vi "UHR-Fleezers Control (host) - 12.0.vi"() -> ()   [LabVIEW 2012] (continued)
            n2040 = Unbundle By Name(w3404) -> ("Set 1"=w3403:dbl, "Set 2"=w3402:dbl)
            n2041 = Unbundle By Name(w3401) -> ("Set 1"=w3400:bool, "Set 2"=w3399:bool)
            n2042 = Select(t=w3397, s=w3400, f=w3403) -> (s? t:f=w3395:dbl)
            n2043 = Select(t=w3396, s=w3399, f=w3402) -> (s? t:f=w3394:dbl)
            n2044 = Bundle By Name(cluster=w3404, "Set 1"=w3395, "Set 2"=w3394) -> (w3392:cluster{"Set 1":dbl, "Set 2":dbl})
            n2045 = local write "Setpoints (V)"(w3392) -> ()
            n2046 = Multiply(x=3276.7, y=w3392) -> (x*y=w3393:cluster{"Set 1":dbl, "Set 2":dbl})
            n2047 = To Word Integer(number=w3393) -> (16bit integer=w3405:cluster{"Set 1":i16, "Set 2":i16})
          }
        }
        n2048 = Unbundle By Name(w3377) -> ("Set 1"=w3376:i16, "Set 2"=w3375:i16)
        n2049 = xnode "Read/Write Control"("FPGA VI Reference In"=w3373, "error in"=w3372, "FB Setpoint Set 1"=w3376, "FB Setpoint Set 2"=w3375) -> ("error out"=w3371:errorcluster)  [unwired: 1 out]
      }
      event "Invert GI": Value Change {
        n2050 = event-data() -> ()  [unwired: 7 out]
        n2051 = xnode "Read/Write Control"("FPGA VI Reference In"=w3410, "error in"=w3408, "Invert GI"="Invert GI", "Invert GI 2"="Invert GI") -> ("error out"=w3409:errorcluster)  [unwired: 1 out]
      }
      event "Green FB Setpoint (mV)", "Green FB Gains", "Green FB On/Off", "Current When FB OFF (%)", "Green int current ON count adj": Value Change {
        n2052 = event-data() -> ()  [unwired: 7 out]
        n2053 = local read "Green FB Setpoint (mV)"() -> (w3417:dbl)
        n2054 = local read "Current When FB OFF (%)"() -> (w3420:dbl)
        n2055 = Multiply(x=w3417, y=3.2767) -> (x*y=w3416:dbl)
        n2056 = Multiply(x=w3420, y=655.35) -> (x*y=w3421:dbl)
        n2057 = To Unsigned Word Integer(number=w3421) -> (unsigned 16bit integer=w3419:u16)
        n2058 = local read "Green int current ON count adj"() -> (w3424:u32)
        n2059 = local read "Green FB Gains"() -> (w3423:T14)
        n2060 = local read "Green Laser ON/Interlacing"() -> (w3414:bool)
        n2061 = local read "Green laser mode"() -> (w3413:enum32{"Laser ON", "Laser OFF", "Interlace"})
        n2062 = local read "Green FB On/Off"() -> (w3425:bool)
        n2063 = Equal?(x=w3413, y=enum32{"Laser ON", "Laser OFF", "Interlace"}."Interlace") -> (x = y?=w3411:bool)
        n2064 = Compound Arithmetic op=AND(w3411, w3425, w3414) -> (w3415:bool)
        n2065 = xnode "Read/Write Control"("FPGA VI Reference In"=w3428, "error in"=w3427, "Green FB Setpoint"=w3416, "Green FB On/Off"=w3415, "Current Out"=w3419, "Green int current ON count adj"=w3424, "Green FB Gains"=w3423) -> ("error out"=w3426:errorcluster)  [unwired: 1 out]
      }
      event "Green laser mode", "Green Laser ON/Interlacing": Value Change {
        n2066 = event-data() -> ()  [unwired: 7 out]
        n2067 = local write "Green Laser ON/OFF"("Green Laser ON/Interlacing") -> ()
        n2068 = case shown="True" "Green Laser ON/Interlacing" {
          tunnel: "Green laser mode" -> [_ w3442]
          tunnel: [enum32{"Laser ON", "Laser OFF", "Interlace"}."Laser OFF" ("Green laser mode") w3442] -> w3431
          tunnel: [FALSE w3438] -> w3430
          frame False {
          }
          frame True {
            n2069 = local read "Green FB On/Off"() -> (w3439:bool)
            n2070 = Equal?(x=w3442, y=enum32{"Laser ON", "Laser OFF", "Interlace"}."Interlace") -> (x = y?=w3440:bool)
            n2071 = And(x=w3440, y=w3439) -> (x .and. y?=w3438:bool)
          }
        }
        n2072 = xnode "Read/Write Control"("FPGA VI Reference In"=w3435, "error in"=w3433, "Operating Mode"=w3431, "Operating Mode 2"=w3431, "Green FB On/Off"=w3430) -> ("error out"=w3434:errorcluster)  [unwired: 1 out]
      }
      event "Green Laser ON/OFF": Value Change {
        n2073 = event-data() -> ()  [unwired: 7 out]
        n2074 = property on="Green Laser ON/Interlacing" class="Bool (strict)"("Val(Sgnl)"="Green Laser ON/OFF") -> ()  [unwired: 2 in, 2 out]
      }
      event "Test ttrig": Value Change {
        n2075 = event-data() -> ()  [unwired: 7 out]
        n2076 = xnode "Read/Write Control"("FPGA VI Reference In"=w3447, "error in"=w3446, "TTrig?"=TRUE) -> ("error out"=w3445:errorcluster)  [unwired: 1 out]
      }
      event "Neg. TTrig FPGA": Value Change {
        n2077 = event-data() -> ()  [unwired: 7 out]
        n2078 = xnode "Read/Write Control"("FPGA VI Reference In"=w3451, "error in"=w3450, "TTrig Negate Pos"="Neg. TTrig FPGA") -> ()  [unwired: 2 out]
      }
      event "- phase (APD 1 Gate)", "+ phase (APD 1 Gate)": Value Change {
        n2079 = event-data() -> ()  [unwired: 7 out]
        n2080 = local read "Phase Adj. (APD 1 Gate)"() -> (w3452:i16)
        n2081 = Negate(x=w3452) -> (-x=w3460:i16)
        n2082 = Select(t=w3460, s="- phase (APD 1 Gate)", f=w3452) -> (s? t:f=w3459:i16)
        n2083 = Or(x="- phase (APD 1 Gate)", y="+ phase (APD 1 Gate)") -> (x .or. y?=w3455:bool)
        n2084 = xnode "Read/Write Control"("FPGA VI Reference In"=w3462, "error in"=w3461, "Phase count adjustment (APD 1 Gate)"=w3459) -> ("FPGA VI Reference Out"=w3457:T19, "error out"=w3458:errorcluster)
        n2085 = xnode "Read/Write Control"("FPGA VI Reference In"=w3457, "error in"=w3458, "+ phase (APD 1 Gate)"=w3455) -> ("error out"=w3456:errorcluster)  [unwired: 1 out]
      }
      event "+ phase (APD 2 Gate)", "- phase (APD 2 Gate)": Value Change {
        n2086 = event-data() -> ()  [unwired: 7 out]
        n2087 = local read "Phase Adj. (APD 2 Gate)"() -> (w3463:i16)
        n2088 = Negate(x=w3463) -> (-x=w3471:i16)
        n2089 = Select(t=w3471, s="- phase (APD 2 Gate)", f=w3463) -> (s? t:f=w3470:i16)
        n2090 = Or(x="- phase (APD 2 Gate)", y="+ phase (APD 2 Gate)") -> (x .or. y?=w3466:bool)
        n2091 = xnode "Read/Write Control"("FPGA VI Reference In"=w3473, "error in"=w3472, "Phase count adjustment (APD 2 Gate)"=w3470) -> ("FPGA VI Reference Out"=w3468:T19, "error out"=w3469:errorcluster)
        n2092 = xnode "Read/Write Control"("FPGA VI Reference In"=w3468, "error in"=w3469, "+ phase (APD 2 Gate)"=w3466) -> ("error out"=w3467:errorcluster)  [unwired: 1 out]
      }
      event "Phase Adj. (APD Acq)", "+ phase (APD Acq)", "- phase (APD Acq)": Value Change {
        n2093 = event-data() -> ()  [unwired: 7 out]
        n2094 = local read "Phase Adj. (APD Acq)"() -> (w3476:i16)
        n2095 = Negate(x=w3476) -> (-x=w3482:i16)
        n2096 = Select(t=w3482, s="+ phase (APD Acq)", f=w3476) -> (s? t:f=w3481:i16)
        n2097 = Or(x="+ phase (APD Acq)", y="- phase (APD Acq)") -> (x .or. y?=w3477:bool)
        n2098 = xnode "Read/Write Control"("FPGA VI Reference In"=w3484, "error in"=w3483, "Phase Count Adjustment (APD Acq)"=w3481) -> ("FPGA VI Reference Out"=w3479:T19, "error out"=w3480:errorcluster)
        n2099 = xnode "Read/Write Control"("FPGA VI Reference In"=w3479, "error in"=w3480, "+ phase (APD Acq)"=w3477) -> ("error out"=w3478:errorcluster)  [unwired: 1 out]
      }
      event "Phase adj. (GI)", "+ phase (GI)", "- phase (GI)": Value Change {
        n2100 = event-data() -> ()  [unwired: 7 out]
        n2101 = Negate(x="Phase adj. (GI)") -> (-x=w3493:i16)
        n2102 = Select(t=w3493, s="+ phase (GI)", f="Phase adj. (GI)") -> (s? t:f=w3492:i16)
        n2103 = Or(x="+ phase (GI)", y="- phase (GI)") -> (x .or. y?=w3488:bool)
        n2104 = xnode "Read/Write Control"("FPGA VI Reference In"=w3495, "error in"=w3494, "Phase count adjustment (GI)"=w3492) -> ("FPGA VI Reference Out"=w3490:T19, "error out"=w3491:errorcluster)
        n2105 = xnode "Read/Write Control"("FPGA VI Reference In"=w3490, "error in"=w3491, "+ phase (GI)"=w3488) -> ("error out"=w3489:errorcluster)  [unwired: 1 out]
      }
      event "Phase adj. (GI) 2", "+ phase (GI) 2", "- phase (GI) 2": Value Change {
        n2106 = event-data() -> ()  [unwired: 7 out]
        n2107 = Negate(x="Phase adj. (GI) 2") -> (-x=w3504:i16)
        n2108 = Select(t=w3504, s="+ phase (GI) 2", f="Phase adj. (GI) 2") -> (s? t:f=w3503:i16)
        n2109 = Or(x="+ phase (GI) 2", y="- phase (GI) 2") -> (x .or. y?=w3499:bool)
        n2110 = xnode "Read/Write Control"("FPGA VI Reference In"=w3506, "error in"=w3505, "Phase count adjustment (GI) 2"=w3503) -> ("FPGA VI Reference Out"=w3501:T19, "error out"=w3502:errorcluster)
        n2111 = xnode "Read/Write Control"("FPGA VI Reference In"=w3501, "error in"=w3502, "+ phase (GI) 2"=w3499) -> ("error out"=w3500:errorcluster)  [unwired: 1 out]
      }
      event "Phase adj. (Green FB)", "- phase (Green FB)", "+ phase (Green FB)": Value Change {
        n2112 = event-data() -> ()  [unwired: 7 out]
        n2113 = Negate(x="Phase adj. (Green FB)") -> (-x=w3515:i16)
        n2114 = Select(t=w3515, s="+ phase (Green FB)", f="Phase adj. (Green FB)") -> (s? t:f=w3514:i16)
        n2115 = Or(x="+ phase (Green FB)", y="- phase (Green FB)") -> (x .or. y?=w3510:bool)
        n2116 = xnode "Read/Write Control"("FPGA VI Reference In"=w3517, "error in"=w3516, "Phase count adjustment (Green FB)"=w3514) -> ("FPGA VI Reference Out"=w3512:T19, "error out"=w3513:errorcluster)
        n2117 = xnode "Read/Write Control"("FPGA VI Reference In"=w3512, "error in"=w3513, "+ phase (Green FB)"=w3510) -> ("error out"=w3511:errorcluster)  [unwired: 1 out]
      }
      event "Invert APD Gate", "APD Gate ON Count", "APD Gate OFF Count", "APD Gate", "APD Integration Time (s)", "APD 1 AO Mult.", "APD 2 AO Mult.", "On one out of X cycles": Value Change {
        n2118 = event-data() -> ()  [unwired: 7 out]
        n2119 = Add(x="GI Frequency, ON count", y="GI Frequency, OFF count") -> (x+y=w3521:u32)
        n2120 = Add(x="APD Gate ON Count", y="APD Gate OFF Count") -> (x+y=w3534:u32)
        n2121 = Multiply(x="On one out of X cycles", y=w3521) -> (x*y=w3518:u32)
        "Green FB Count" <- w3518
        n2122 = Subtract(x=w3518, y="GI Frequency, ON count") -> (x-y=w3519:u32)
        n2123 = Multiply(x=w3534, y="On one out of X cycles") -> (x*y=w3533:u32)
        n2124 = Subtract(x=w3533, y="APD Gate ON Count") -> (x-y=w3532:u32)
        n2125 = local read "DMA Update Period (s)"() -> (w3535:dbl)
        n2126 = Multiply(x="APD Integration Time (s)", y=40000000.0) -> (x*y=w3540:dbl)
        n2127 = Reciprocal(x="APD Integration Time (s)") -> (1/x=→"APD Acq Rate (Hz)":dbl)
        n2128 = To Unsigned Long Integer(number=w3540) -> (unsigned 32bit integer=w3524:u32)
        "APD Int. Count" <- w3524
        n2129 = xnode "Read/Write Control"("FPGA VI Reference In"=w3544, "error in"=w3543, "Invert APD Gate"="Invert APD Gate", "APD Gate ON Count"="APD Gate ON Count", "APD Gate OFF Count"=w3532, "APD Acq Rate Count"=w3524, "APD Gate Operating Mode"="APD Gate", "APD 1 AO scale factor"="APD 1 AO Mult.", "APD 2 AO scale factor"="APD 2 AO Mult.", "Green interlace ON count"="GI Frequency, ON count", "Green interlace OFF count"=w3519, "Green interlace ON count 2"="GI Frequency, ON count", "Green interlace OFF count 2"=w3519, "Green FB Count"=w3518) -> ("error out"=w3542:errorcluster)  [unwired: 1 out]
        n2130 = Divide(x=w3535, y="APD Integration Time (s)") -> (x/y=w3538:dbl)
        n2131 = Multiply(x=2.0, y=w3538) -> (x*y=w3537:dbl)
        n2132 = local write "APD Samples/FIFO Acq."(w3538) -> ()
        n2133 = local write "APD Elements/DMA read"(w3537) -> ()
      }
      event "Number of F/B Scans (AOD)", "Scan Speed (nm/s)", "Scan BD", "Initial delta (MHz)", "Step Size (nm)", "Scan Range (nm)": Value Change {
        w3606 = 123.0  # AOM cal (nm/MHz)
        n2134 = event-data() -> ()  [unwired: 7 out]
        n2135 = local read "BD 1 Frequency 1 (MHz)"() -> (w3589:dbl)
        n2136 = local read "AOM X Cal (nm/MHz)"() -> (w3581:dbl)
        n2137 = local read "X RF Frequency Limits (MHz)"() -> (w3593:T16)
        n2138 = local read "Y RF Frequency Limits (MHz)"() -> (w3590:T16)
        n2139 = local read "BD 2 Frequency 1 (MHz)"() -> (w3595:dbl)
        n2140 = Negate(x="Scan Range (nm)") -> (-x=w3559:dbl)
        n2141 = Divide(x=w3559, y=w3581) -> (x/y=w3563:dbl)
        n2142 = Select(t=w3593, s="Scan BD", f=w3590) -> (s? t:f=w3592:T16)
        n2143 = Select(t=w3589, s="Scan BD", f=w3595) -> (s? t:f=w3594:dbl)
        n2144 = Unbundle By Name(w3592) -> ("Maximum"=w3601:dbl, "Minimum"=w3600:dbl)
        n2145 = Add(x=w3563, y=w3594) -> (x+y=w3598:dbl)
        n2146 = Divide(x=w3559, y="Step Size (nm)") -> (x/y=w3578:dbl)
        n2147 = Divide(x="Step Size (nm)", y=w3581) -> (x/y=w3587:dbl)
        n2148 = Absolute Value(x=w3578) -> (abs(x)=w3562:dbl)
        n2149 = Sign(1:w3559) -> (0:w3560:dbl)
        n2150 = In Range and Coerce(upper limit=w3601, x=w3598, lower limit=w3600) -> (coerced(x)=w3597:dbl, In Range?=w3599:bool)
        n2151 = To Unsigned Quad Integer(1:w3562) -> (0:w3577:u64)
        "Scan steps (AOD)" <- w3577
        n2152 = call "IR AOM freq to word.vi"("Frequency In (MHz)"=w3587) -> ("Frequency Word Out (double)"=w3584:dbl)
        n2153 = Multiply(x=w3560, y=w3584) -> (x*y=w3561:dbl)
        n2154 = Subtract(x=w3598, y=w3597) -> (x-y=w3596:dbl)
        n2155 = To Quad Integer(1:w3561) -> (0:w3583:i64)
        "Incr. int (AOD)" <- w3583
        n2156 = Subtract(x=w3563, y=w3596) -> (x-y=w3582:dbl)
        "Scan Range (MHz)" <- w3582
        n2157 = Select(t=w3563, s=w3599, f=w3582) -> (s? t:f=w3602:dbl)
        n2158 = Multiply(x=w3582, y=w3581) -> (x*y=w3580:dbl)
        n2159 = Decrement(x=w3577) -> (x-1=w3630:u64)
        n2160 = Negate(x=w3580) -> (-x=w3576:dbl)
        n2161 = local write "Scan Range (nm)"(w3576) -> ()
        n2162 = Divide(x=w3602, y=w3630) -> (x/y=w3586:dbl)
        "Scan Increment (MHz)" <- w3586
        n2163 = call "IR AOM freq to word.vi"("Frequency In (MHz)"=w3586) -> ("Frequency Word Out (double)"=w3585:dbl)
        n2164 = Divide(x="Step Size (nm)", y="Scan Speed (nm/s)") -> (x/y=w3573:dbl)
        n2165 = To Quad Integer(1:w3585) -> ()  [unwired: 1 out]
        n2166 = local read "Number Interlace Sets"() -> (w3557:u8)
        n2167 = local read "AI Count (ticks)"() -> (w3558:u32)
        n2168 = local read "Total Counts (ticks)"() -> (w3556:u32)
        n2169 = local read "# Samples/trap"() -> (w3588:u32)
        n2170 = Multiply(x=w3558, y=w3557) -> (x*y=w3555:u32)
        n2171 = Divide(x=w3556, y=w3555) -> (x/y=w3554:dbl)
        n2172 = Select(t=w3589, s="Scan BD", f=w3595) -> (s? t:f=w3627:dbl)
        "Initial freq. (MHz)" <- w3627
        n2173 = Add(x=w3602, y=w3627) -> (x+y=→"Final freq. (MHz)":dbl)
        n2174 = Divide(x=w3556, y=40000000.0) -> (x/y=w3572:dbl)
        n2175 = Divide(x=w3573, y=w3572) -> (x/y=w3571:dbl)
        n2176 = To Unsigned Quad Integer(1:w3571) -> (0:w3546:u64)
        n2177 = Quotient & Remainder(x=w3546, y=u64 2) -> (x-y*floor(x/y)=w3550:u64)  [unwired: 1 out]
        n2178 = Equal?(x=w3550, y=u64 0) -> (x = y?=w3548:bool)
        n2179 = Decrement(x=w3546) -> (x-1=w3547:u64)
        n2180 = Select(t=w3546, s=w3548, f=w3547) -> (s? t:f=w3545:u64)
        "Cycles/step (AOD)" <- w3545
        n2181 = xnode "Read/Write Control"("FPGA VI Reference In"=w3638, "error in"=w3637, "Scan steps"=w3577, "Number of scans"="Number of F/B Scans (AOD)", "Cycles per step"=w3545, "Scan freq.  increment"=w3583, "Scan BD"="Scan BD") -> ("error out"=w3636:errorcluster)  [unwired: 1 out]
        n2182 = Multiply(x=w3577, y=w3545) -> (x*y=w3631:u64)
        n2183 = Multiply(x=w3631, y=u64 2) -> (x*y=w3553:u64)
        n2184 = Multiply(x=w3554, y=w3553) -> (x*y=w3552:dbl)
        "Data points/scan (f/b)" <- w3552
        n2185 = Multiply(x=w3552, y="Number of F/B Scans (AOD)") -> (x*y=w3634:dbl)
        "Data points/scans" <- w3634
        n2186 = Divide(x=w3634, y=w3588) -> (x/y=→"N sets should be saved":dbl)
        n2187 = Multiply(x=w3631, y=w3572) -> (x*y=w3570:dbl)
        "Time/Scan (s) (AOD)" <- w3570
        n2188 = Select(t=w3602, s="Scan BD", f=0.0) -> (s? t:f=w3628:dbl)
        n2189 = Select(t=0.0, s="Scan BD", f=w3602) -> (s? t:f=w3624:dbl)
        n2190 = local read "BD 2 Frequency 2 (MHz)"() -> (w3620:dbl)
        n2191 = local read "BD 1 Frequency 2 (MHz)"() -> (w3623:dbl)
        n2192 = Add(x=w3624, y=w3595) -> (x+y=w3621:dbl)
        n2193 = Add(x=w3589, y=w3628) -> (x+y=w3622:dbl)
        n2194 = Multiply(x=w3570, y=2.0) -> (x*y=w3569:dbl)
        n2195 = Multiply(x=w3569, y="Number of F/B Scans (AOD)") -> (x*y=w3566:dbl)
        n2196 = Divide(x=w3566, y=60.0) -> (x/y=→"Time to Finish All (min)":dbl)
        n2197 = Add(x="Trap 2 Bead Size (nm)", y="Trap 1 Bead Size (nm)") -> (x+y=w3610:dbl)
        n2198 = Divide(x=w3610, y=2.0) -> (x/y=w3604:dbl)
        n2199 = local read "Initial delta (MHz)"() -> (w3607:dbl)
        n2200 = Subtract(x=w3621, y=w3620) -> (x-y=w3618:dbl)
        n2201 = Subtract(x=w3622, y=w3623) -> (x-y=w3619:dbl)
        n2202 = Square(x=w3618) -> (x^2=w3617:dbl)
        n2203 = Square(x=w3619) -> (x^2=w3616:dbl)
        n2204 = Add(x=w3616, y=w3617) -> (x+y=w3615:dbl)
        n2205 = Square Root(x=w3615) -> (sqrt(x)=w3614:dbl)
        "Final delta (MHz)" <- w3614
        n2206 = Multiply(x=w3606, y=w3614) -> (x*y=w3613:dbl)
        n2207 = Multiply(x=w3607, y=w3606) -> (x*y=w3605:dbl)
        n2208 = Subtract(x=w3605, y=w3604) -> (x-y=→"Initial sep (nm)":dbl)
        n2209 = Subtract(x=w3613, y=w3604) -> (x-y=→"Final sep (nm)":dbl)
      }
      event "Freq or Amp switch first", "Swap F1 and F2", "Freq switch delay", "Amp switch delay": Value Change {
        n2210 = event-data() -> ()  [unwired: 7 out]
        n2211 = local read "Freq or Amp switch first"() -> (w3639:bool)
        n2212 = local read "Amp switch delay"() -> (w3640:u16)
        n2213 = local read "Freq switch delay"() -> (w3642:u16)
        n2214 = local read "Swap F1 and F2"() -> (w3641:bool)
        n2215 = xnode "Read/Write Control"("FPGA VI Reference In"=w3645, "error in"=w3644, "Freq switch delay"=w3642, "Swap F1 and F2"=w3641, "Amp switch delay"=w3640, "Freq or Amp switch first"=w3639) -> ("error out"=w3643:errorcluster)  [unwired: 1 out]
      }
      event "Scan steps (MCL)", "Number of scans (MCL)", "Scan Range (V)\n(of steps)", "2D or 1D Scan", "N APD Samp/step", "Fast Scan Dir", "Continuous MCL Scanning", "Scan lines (y)": Value Change {
        w3647 = 32767.0 ("y")
        n2216 = event-data() -> ()  [unwired: 7 out]
        n2217 = Select(t="Scan lines (y)", s="2D or 1D Scan", f="Number of scans (MCL)") -> (s? t:f=w3652:u64)
        n2218 = Decrement(x="Scan steps (MCL)") -> (x-1=w3668:u64)
        n2219 = Divide(x="Scan Range (V)\n(of steps)", y=w3668) -> (x/y=w3667:dbl)
        "Desired Scan Incr (V)" <- w3667
        n2220 = local read "APD Integration Time (s)"() -> (w3660:dbl)
        n2221 = Multiply(x=w3667, y=w3647) -> (x*y=w3676:dbl)
        n2222 = Divide(x=w3676, y=10.0) -> (x/y=w3666:dbl)
        "Desired incr (int)" <- w3666
        n2223 = local read "Update Count (MCL)"() -> (w3672:u32)
        n2224 = Round Toward -Infinity(1:w3666) -> (0:w3675:dbl)
        n2225 = To Word Integer(number=w3675) -> (16bit integer=w3650:i16)
        "Actual Incr. int (MCL)" <- w3650
        n2226 = Multiply(x=w3660, y=40000000.0) -> (x*y=w3673:dbl)
        n2227 = Divide(x=w3673, y=w3672) -> (x/y=w3671:dbl)
        n2228 = Multiply(x=i16 10, y=w3650) -> (x*y=w3648:i16)
        n2229 = Multiply(x="N APD Samp/step", y=w3671) -> (x*y=w3670:dbl)
        "Cycles/step (MCL)" <- w3670
        n2230 = Divide(x=w3648, y=w3647) -> (x/y=→"Actual MCL Inc (V)":dbl)
        n2231 = Multiply(x="N APD Samp/step", y="Scan steps (MCL)") -> (x*y=w3662:dbl)
        n2232 = local read "APD Samples/FIFO Acq."() -> (w3659:dbl)
        n2233 = Multiply(x=w3662, y=u64 2) -> (x*y=w3661:dbl)
        "Data points/scan (f+b)" <- w3661
        n2234 = Multiply(x=w3661, y=w3652) -> (x*y=w3679:dbl)
        "Data points/scans (MCL)" <- w3679
        n2235 = Multiply(x=w3660, y=w3661) -> (x*y=w3653:dbl)
        "Time/f+b scan (s) (MCL)" <- w3653
        n2236 = Divide(x=w3679, y=w3659) -> (x/y=→"N sets should be saved (MCL)":dbl)
        n2237 = Multiply(x=w3653, y=w3652) -> (x*y=→"Total Time (s)":dbl)
        n2238 = Not(x="Fast Scan Dir") -> (.not. x?=w3657:bool)
        n2239 = xnode "Read/Write Control"("FPGA VI Reference In"=w3683, "error in"=w3682, "Scan steps (MCL)"="Scan steps (MCL)", "Number of scans (MCL)"=w3652, "Cycles per step (MCL)"=w3670, "Scan freq.  increment (MCL)"=w3650, "1D or 2D Scan?"="2D or 1D Scan", "MCL Scan Axis"=w3657, "Cont. Scan (MCL)"="Continuous MCL Scanning") -> ("error out"=w3681:errorcluster)  [unwired: 1 out]
      }
      event "Read Cal": Value Change {
        w3685 = 1000.0 ("y")
        n2240 = event-data() -> ()  [unwired: 7 out]
        n2241 = local read "Save file name"() -> (w3710:path)
        n2242 = local write "Read Cal"(FALSE ("Read Cal")) -> ()
        n2243 = Strip Path(path=w3710) -> (stripped path=w3709:path)  [unwired: 1 out]
        n2244 = Path To String(path=w3709) -> (string=w3708:string)
        n2245 = Concatenate Strings(w3708, "\\current.cal" ("string")) -> (w3706:string)
        n2246 = String To Path(string=w3706) -> (path=w3705:path)
        n2247 = Open/Create/Replace File(file path (use dialog)=w3705, operation (0:open)=T35."open", access (0:read/write)=enum16{"read/write", "read-only", "write-only"}."read-only") -> (refnum out=w3713:refnum<file>, error out=w3699:errorcluster)  [unwired: 1 in, 3 out]
        n2248 = Deny Access(4:w3699, 7:w3713) -> (0:w3698:errorcluster, 3:w3704:refnum<file>)  [unwired: 1 out]
        n2249 = Read from Binary File(5:0.0, 8:w3698, 9:T36."big-endian, network order" ("byte order (0:big-endian, network order)"), 10:-1 ("count (1)"), 11:w3704) -> (0:w3697:errorcluster, 2:w3695:dbl[], 3:w3700:refnum<file>)  [unwired: 2 out]
        n2250 = Array To Cluster(array=w3695) -> (cluster=w3694:T44)
        n2251 = Unbundle(w3694) -> ("[0]"=w3693:dbl, "[1]"=w3692:dbl, "[2]"=w3691:dbl, "[3]"=w3690:dbl, "[4]"=w3689:dbl, "[5]"=w3688:dbl)
        n2252 = Close File(refnum=w3700, error in=w3697) -> (error out=→"Read cal error":errorcluster)  [unwired: 1 out]
        n2253 = Multiply(x=w3688, y=w3685) -> (x*y=w3686:dbl)
        n2254 = local write "T2 kappa_x (pN/nm)"(w3690) -> ()
        n2255 = local write "T1 kappa_x (pN/nm)"(w3691) -> ()
        n2256 = local write "T1 alpha_x (nm/V)"(w3693) -> ()
        n2257 = local write "T2 alpha_x (nm/V)"(w3692) -> ()
        n2258 = Multiply(x=w3689, y=w3685) -> (x*y=w3687:dbl)
        n2259 = local write "T1 offset_x (mV)"(w3687) -> ()
        n2260 = local write "T2 offset_x (mV)"(w3686) -> ()
      }
      event "Abort MCL Scan": Value Change {
        n2261 = event-data() -> ()  [unwired: 7 out]
        n2262 = local write "MCL Scanning"(FALSE ("MCL Scanning")) -> ()
        n2263 = xnode "Read/Write Control"("FPGA VI Reference In"=w3718, "error in"=w3717, "Abort scan (MCL)"="Abort MCL Scan") -> ("error out"=w3716:errorcluster)  [unwired: 1 out]
      }
      event "Update Count (MCL)": Value Change {
        n2264 = event-data() -> ()  [unwired: 7 out]
        n2265 = xnode "Read/Write Control"("FPGA VI Reference In"=w3722, "error in"=w3721, "MCL count"="Update Count (MCL)") -> ("error out"=w3720:errorcluster)  [unwired: 1 out]
      }
      event "Phase adjust (MCL)", "+ phase (MCL)", "- phase (MCL)": Value Change {
        n2266 = event-data() -> ()  [unwired: 7 out]
        n2267 = Negate(x="Phase adjust (MCL)") -> (-x=w3731:i16)
        n2268 = Select(t=w3731, s="- phase (MCL)", f="Phase adjust (MCL)") -> (s? t:f=w3729:i16)
        n2269 = Or(x="- phase (MCL)", y="+ phase (MCL)") -> (x .or. y?=w3724:bool)
        n2270 = xnode "Read/Write Control"("FPGA VI Reference In"=w3733, "error in"=w3732, "Phase count adjustment (MCL)"=w3729) -> ("FPGA VI Reference Out"=w3725:T19, "error out"=w3726:errorcluster)
        n2271 = xnode "Read/Write Control"("FPGA VI Reference In"=w3725, "error in"=w3726, "+ phase (MCL)"=w3724) -> ("error out"=w3723:errorcluster)  [unwired: 1 out]
      }
      event "Abort AOD Scan": Value Change {
        n2272 = event-data() -> ()  [unwired: 7 out]
        n2273 = xnode "Read/Write Control"("FPGA VI Reference In"=w3737, "error in"=w3736, "Abort scan"="Abort AOD Scan") -> ("error out"=w3735:errorcluster)  [unwired: 1 out]
      }
      event "Continuous AOD Scanning": Value Change {
        n2274 = event-data() -> ()  [unwired: 7 out]
        n2275 = xnode "Read/Write Control"("FPGA VI Reference In"=w3741, "error in"=w3740, "Cont. Scan"="Continuous AOD Scanning") -> ("error out"=w3739:errorcluster)  [unwired: 1 out]
      }
      event "Index": Value Change {
        n2276 = event-data() -> ()  [unwired: 7 out]
        n2277 = call "Create new save file.vi"("Insert"="", "Ext"=".dat" ("string"), "Index In"="Index") -> ("Path Out"=→"Save file name":path, "Index Out"=w3742:dbl)
        "Save index" <- w3742
        n2278 = local write "Index"(w3742) -> ()
      }
      event "AO1", "AO2": Value Change {
        w3757 = 10.0 ("y")
        w3756 = 32767.0 ("y")
        n2279 = event-data() -> ()  [unwired: 7 out]
        n2280 = local read "AO2"() -> (w3755:dbl)
        n2281 = local read "AO1"() -> (w3752:dbl)
        n2282 = Multiply(x=w3752, y=w3756) -> (x*y=w3751:dbl)
        n2283 = Multiply(x=w3755, y=w3756) -> (x*y=w3754:dbl)
        n2284 = Divide(x=w3751, y=w3757) -> (x/y=w3750:dbl)
        n2285 = Divide(x=w3754, y=w3757) -> (x/y=w3753:dbl)
        n2286 = To Word Integer(number=w3750) -> (16bit integer=w3758:i16)
        n2287 = To Word Integer(number=w3753) -> (16bit integer=w3759:i16)
        n2288 = xnode "Read/Write Control"("FPGA VI Reference In"=w3749, "error in"=w3748, "AO1"=w3758, "AO2"=w3759) -> ("error out"=w3747:errorcluster)  [unwired: 1 out]
      }
      event "Inject Pump 1": Value Change {
        n2289 = event-data() -> ()  [unwired: 7 out]
        n2290 = local read "Use Harvard pumps\nfor beads (else Chemyx)"() -> (w3761:bool)
        n2291 = case shown="True" w3761 {
          tunnel: "Inject Pump 1" -> [w3765 w3803]
          tunnel: w3760 -> [_ w3804]
          frame False {
            n2292 = local read "Pump write delay (ms)"() -> (w3764:dbl)
            n2293 = local read "Chemyx Syringe Pump Serial Port"() -> (w3763:refnum<visa-resource-name>)
            n2294 = case shown="True" w3765 {
              tunnel: w3764 -> [w3771 w3785]
              tunnel: w3763 -> [w3768 w3784]
              frame False {
                n2295 = flat-sequence {
                  tunnel: w3768 -> [w3772]
                  tunnel: [w3772] -> w3769
                  tunnel: w3771 -> [_]
                  tunnel: [w3775] -> w3770
                  tunnel: w3769 -> [w3775]
                  tunnel: w3770 -> [w3776]
                  tunnel: [w3776] -> w3766
                  tunnel: [w3778] -> w3767
                  tunnel: w3766 -> [w3778]
                  tunnel: w3767 -> [w3780]
                  frame #0 {
                    n2296 = call "Write to pump.vi"("string"="enter pump1", "VISA resource name"=w3772) -> ()  [unwired: 1 out]
                  }
                  frame #1 {
                    n2297 = Wait (ms)(milliseconds to wait="Pump pause delay (ms)") -> ()  [unwired: 1 out]
                  }
                  frame #2 {
                    n2298 = call "Write to pump.vi"("string"="stop", "VISA resource name"=w3776) -> ()  [unwired: 1 out]
                  }
                  frame #3 {
                    n2299 = Wait (ms)(milliseconds to wait=u32 500) -> ()  [unwired: 1 out]
                  }
                  frame #4 {
                    n2300 = call "Write to pump.vi"("string"="stop", "VISA resource name"=w3780) -> ()  [unwired: 1 out]
                  }
                }
              }
              frame True {
                n2301 = flat-sequence {
                  tunnel: w3784 -> [w3794]
                  tunnel: w3785 -> [w3789]
                  tunnel: w3785 -> [w3796]
                  tunnel: w3784 -> [w3797]
                  tunnel: [w3797] -> w3782
                  tunnel: [w3799] -> w3783
                  tunnel: w3782 -> [w3799]
                  tunnel: w3783 -> [w3801]
                  frame #0 {
                    n2302 = local read "All Pump Parameters"() -> (w3788:T5)
                    n2303 = Unbundle By Name(w3788) -> ("Pump 1"=w3795:T45)
                    n2304 = call "Set pump parameters.vi"("Pump write delay (ms)"=w3789, "Volume (uL)"="Ch 1 Inject Volume (uL)", "Rate (uL/h)"="Ch 1 Inject Rate (ul/h)", "Units"=4.0, "Pump #"=1.0, "Pump Parameters In"=w3795, "VISA resource name"=w3794) -> ("Pump Parameters Out"=w3787:T45)  [unwired: 3 in]
                    n2305 = Bundle By Name(cluster=w3788, "Pump 1"=w3787) -> (w3786:T5)
                    n2306 = local write "All Pump Parameters"(w3786) -> ()
                  }
                  frame #1 {
                    n2307 = Wait (ms)(milliseconds to wait=w3796) -> ()  [unwired: 1 out]
                  }
                  frame #2 {
                    n2308 = call "Write to pump.vi"("string"="start", "VISA resource name"=w3797) -> ()  [unwired: 1 out]
                  }
                  frame #3 {
                    n2309 = Wait (ms)(milliseconds to wait=u32 500) -> ()  [unwired: 1 out]
                  }
                  frame #4 {
                    n2310 = call "Write to pump.vi"("string"="start", "VISA resource name"=w3801) -> ()  [unwired: 1 out]
                  }
                }
              }
            }
          }
          frame True {
            n2311 = case shown="False" w3803 {
              tunnel: w3804 -> [w3805 w3815]
              frame False {
                n2312 = flat-sequence {
                  tunnel: w3805 -> [w3807]
                  frame #0 {
                    n2313 = local write "Flushing P1"(FALSE ("Flushing P1")) -> ()
                    n2314 = Concatenate Strings("stop" ("string"), "\r") -> (w3809:string)
                    n2315 = VISA Write(VISA resource name=w3807, write buffer=w3809) -> ()  [unwired: 1 in, 3 out]
                  }
                  frame #1 {
                    n2316 = property on="Clear Volume P1" class="Bool (strict)"("Val(Sgnl)"=TRUE ("Value (Signaling)")) -> ()  [unwired: 2 in, 2 out]
                  }
                }
              }
              frame True {
                n2317 = local read "Normal Flow Rate (ul/h) P1"() -> (w3813:dbl)
                n2318 = Number To Decimal String(number=w3813) -> (decimal integer string=w3819:string)  [unwired: 1 in]
                n2319 = Concatenate Strings("irate  " ("string"), w3819, " u/h" ("string"), "\r") -> (w3817:string)
                n2320 = VISA Write(VISA resource name=w3815, write buffer=w3817) -> (VISA resource name out=w3814:refnum<visa-resource-name>)  [unwired: 1 in, 2 out]
                n2321 = Concatenate Strings("irun" ("string"), "\r") -> (w3821:string)
                n2322 = VISA Write(VISA resource name=w3814, write buffer=w3821) -> ()  [unwired: 1 in, 3 out]
              }
            }
          }
        }
      }
      event "Inject Pump 3": Value Change {
        n2323 = event-data() -> ()  [unwired: 7 out]
        n2324 = local read "Use Harvard pumps\nfor beads (else Chemyx)"() -> (w3824:bool)
        n2325 = case shown="True" w3824 {
          tunnel: "Inject Pump 3" -> [w3828 w3867]
          tunnel: w3823 -> [_ w3866]
          frame False {
            n2326 = local read "Pump write delay (ms)"() -> (w3827:dbl)
            n2327 = case shown="True" w3828 {
              tunnel: w3827 -> [w3834 w3848]
              tunnel: "Chemyx Syringe Pump Serial Port" -> [w3831 w3847]
              frame False {
                n2328 = flat-sequence {
                  tunnel: w3831 -> [w3835]
                  tunnel: [w3835] -> w3832
                  tunnel: w3834 -> [_]
                  tunnel: [w3838] -> w3833
                  tunnel: w3832 -> [w3838]
                  tunnel: w3833 -> [w3839]
                  tunnel: [w3839] -> w3829
                  tunnel: [w3841] -> w3830
                  tunnel: w3829 -> [w3841]
                  tunnel: w3830 -> [w3843]
                  frame #0 {
                    n2329 = call "Write to pump.vi"("string"="enter pump3", "VISA resource name"=w3835) -> ()  [unwired: 1 out]
                  }
                  frame #1 {
                    n2330 = local read "Pump pause delay (ms)"() -> (w3837:u32)
                    n2331 = Wait (ms)(milliseconds to wait=w3837) -> ()  [unwired: 1 out]
                  }
                  frame #2 {
                    n2332 = call "Write to pump.vi"("string"="stop", "VISA resource name"=w3839) -> ()  [unwired: 1 out]
                  }
                  frame #3 {
                    n2333 = Wait (ms)(milliseconds to wait=u32 0) -> ()  [unwired: 1 out]
                  }
                  frame #4 {
                    n2334 = call "Write to pump.vi"("string"="stop", "VISA resource name"=w3843) -> ()  [unwired: 1 out]
                  }
                }
              }
              frame True {
                n2335 = flat-sequence {
                  tunnel: w3847 -> [w3857]
                  tunnel: w3848 -> [w3852]
                  tunnel: w3848 -> [w3859]
                  tunnel: w3847 -> [w3860]
                  tunnel: [w3860] -> w3846
                  tunnel: [w3863] -> w3845
                  tunnel: w3846 -> [w3863]
                  tunnel: w3845 -> [w3864]
                  frame #0 {
                    n2336 = local read "All Pump Parameters"() -> (w3851:T5)
                    n2337 = Unbundle By Name(w3851) -> ("Pump 3"=w3858:T45)
                    n2338 = call "Set pump parameters.vi"("Pump write delay (ms)"=w3852, "Volume (uL)"="Ch 3 Inject Volume (uL)", "Rate (uL/h)"="Ch 3 Inject Rate (ul/h)", "Units"=4.0, "Pump #"=3.0, "Pump Parameters In"=w3858, "VISA resource name"=w3857) -> ("Pump Parameters Out"=w3850:T45)  [unwired: 3 in]
                    n2339 = Bundle By Name(cluster=w3851, "Pump 3"=w3850) -> (w3849:T5)
                    n2340 = local write "All Pump Parameters"(w3849) -> ()
                  }
                  frame #1 {
                    n2341 = Wait (ms)(milliseconds to wait=w3859) -> ()  [unwired: 1 out]
                  }
                  frame #2 {
                    n2342 = call "Write to pump.vi"("string"="start", "VISA resource name"=w3860) -> ()  [unwired: 1 out]
                  }
                  frame #3 {
                    n2343 = Wait (ms)(milliseconds to wait=u32 500) -> ()  [unwired: 1 out]
                  }
                  frame #4 {
                    n2344 = call "Write to pump.vi"("string"="start", "VISA resource name"=w3864) -> ()  [unwired: 1 out]
                  }
                }
              }
            }
          }
          frame True {
            n2345 = case shown="False" w3867 {
              tunnel: w3866 -> [w3868 w3875]
              frame False {
                n2346 = flat-sequence {
                  tunnel: w3868 -> [w3870]
                  frame #0 {
                    n2347 = local write "Flushing P3"(FALSE ("Flushing P3")) -> ()
                    n2348 = Concatenate Strings("stop" ("string"), "\r") -> (w3872:string)
                    n2349 = VISA Write(VISA resource name=w3870, write buffer=w3872) -> ()  [unwired: 1 in, 3 out]
                  }
                  frame #1 {
                    n2350 = property on="Clear Volume P3" class="Bool (strict)"("Val(Sgnl)"=TRUE ("Value (Signaling)")) -> ()  [unwired: 2 in, 2 out]
                  }
                }
              }
              frame True {
                n2351 = local read "Normal Flow Rate (ul/h) P3"() -> (w3876:dbl)
                n2352 = Number To Decimal String(number=w3876) -> (decimal integer string=w3882:string)  [unwired: 1 in]
                n2353 = Concatenate Strings("irate  " ("string"), w3882, " u/h" ("string"), "\r") -> (w3880:string)
                n2354 = VISA Write(VISA resource name=w3875, write buffer=w3880) -> (VISA resource name out=w3878:refnum<visa-resource-name>)  [unwired: 1 in, 2 out]
                n2355 = Concatenate Strings("irun" ("string"), "\r") -> (w3884:string)
                n2356 = VISA Write(VISA resource name=w3878, write buffer=w3884) -> ()  [unwired: 1 in, 3 out]
              }
            }
          }
        }
      }
      event "Inject Pump 2": Value Change {
        n2357 = event-data() -> ()  [unwired: 7 out]
        n2358 = local read "Pump write delay (ms)"() -> (w3888:dbl)
        n2359 = flat-sequence {
          tunnel: w3886 -> [w3901]
          tunnel: w3888 -> [w3897]
          tunnel: "Inject Pump 2" -> [_]
          tunnel: w3888 -> [w3903]
          tunnel: w3886 -> [w3904]
          frame #0 {
            n2360 = local read "All Pump Parameters"() -> (w3896:T5)
            n2361 = Multiply(x=60.0, y="Flush Center Ch Rate (ul/m)") -> (x*y=w3893:dbl)
            n2362 = Unbundle By Name(w3896) -> ("Pump 2"=w3902:T45)
            n2363 = call "Set pump parameters.vi"("Pump write delay (ms)"=w3897, "Volume (uL)"="Flush Center Ch Volume (uL)", "Rate (uL/h)"=w3893, "Units"=3.0, "Pump #"=2.0, "Pump Parameters In"=w3902, "VISA resource name"=w3901) -> ("Pump Parameters Out"=w3895:T45)  [unwired: 3 in]
            n2364 = Bundle By Name(cluster=w3896, "Pump 2"=w3895) -> (w3894:T5)
            n2365 = local write "All Pump Parameters"(w3894) -> ()
            n2366 = Add(x="Flush Center Ch Volume (uL)", y="Total Volume\nFlushed (uL)") -> (x+y=w3890:dbl)
            n2367 = local write "Total Volume\nFlushed (uL)"(w3890) -> ()
          }
          frame #1 {
            n2368 = Wait (ms)(milliseconds to wait=w3903) -> ()  [unwired: 1 out]
          }
          frame #2 {
            n2369 = call "Write to pump.vi"("string"="start", "VISA resource name"=w3904) -> ()  [unwired: 1 out]
          }
        }
        n2370 = local read "Chemyx Syringe Pump Serial Port"() -> (w3886:refnum<visa-resource-name>)
      }
      event "Sample Channel\nFlow": Value Change {
        n2371 = event-data() -> ()  [unwired: 7 out]
        n2372 = Select(t="irun" ("string"), s="Sample Channel\nFlow", f="stop" ("string")) -> (s? t:f=w3908:string)
        n2373 = Concatenate Strings(w3908, "\r") -> (w3911:string)
        n2374 = VISA Write(VISA resource name=w3906, write buffer=w3911) -> ()  [unwired: 1 in, 3 out]
      }
      event "Start Flow": Value Change {
        n2375 = event-data() -> ()  [unwired: 7 out]
        n2376 = local write "Sample Channel\nFlow"(TRUE ("Sample Channel\nFlow")) -> ()
        n2377 = local write "Start Flow"(FALSE ("Start Flow")) -> ()
        n2378 = Concatenate Strings("irun" ("string"), "\r") -> (w3917:string)
        n2379 = VISA Write(VISA resource name=w3913, write buffer=w3917) -> ()  [unwired: 1 in, 3 out]
      }
      event "Stop Flow": Value Change {
        w3919 = FALSE ("Stop Flow")
        n2380 = event-data() -> ()  [unwired: 7 out]
        n2381 = local write "Stop Flow"(w3919) -> ()
        n2382 = local write "Sample Channel\nFlow"(w3919) -> ()
        n2383 = Concatenate Strings("stop" ("string"), "\r") -> (w3922:string)
        n2384 = VISA Write(VISA resource name=w3920, write buffer=w3922) -> ()  [unwired: 1 in, 3 out]
      }
      event "Flow rate (uL/h)": Value Change {
        n2385 = event-data() -> ()  [unwired: 7 out]
        n2386 = Number To Decimal String(number="Flow rate (uL/h)") -> (decimal integer string=w3929:string)  [unwired: 1 in]
        n2387 = Concatenate Strings("irate  " ("string"), w3929, " u/h" ("string"), "\r") -> (w3928:string)
        n2388 = VISA Write(VISA resource name=w3925, write buffer=w3928) -> ()  [unwired: 1 in, 3 out]
      }
      event "Flush Sample": Value Change {
        n2389 = event-data() -> ()  [unwired: 7 out]
        n2390 = flat-sequence {
          tunnel: w3934 -> [w3962]
          tunnel: [w3942] -> w3933
          tunnel: [w3936] -> w3931
          tunnel: w3933 -> [w3966]
          tunnel: [w3966] -> w3932
          tunnel: w3931 -> [w3965]
          tunnel: w3932 -> [w3971]
          frame #0 {
            # "set paramaters (rate, volume) for flush, clear volume"
            n2391 = Number To Decimal String(number="Flush rate (uL/m)") -> (decimal integer string=w3958:string)  [unwired: 1 in]
            n2392 = Concatenate Strings("irate  " ("string"), w3958, " u/m" ("string"), "\r") -> (w3960:string)
            n2393 = VISA Write(VISA resource name=w3962, write buffer=w3960) -> (VISA resource name out=w3956:refnum<visa-resource-name>)  [unwired: 1 in, 2 out]
            n2394 = Reciprocal(x="Flush rate (uL/m)") -> (1/x=w3939:dbl)
            n2395 = Number To Decimal String(number="Volume (uL)") -> (decimal integer string=w3947:string)  [unwired: 1 in]
            n2396 = Multiply(x="Volume (uL)", y=w3939) -> (x*y=w3938:dbl)
            n2397 = Concatenate Strings("tvolume  " ("string"), w3947, " u" ("string"), "\r") -> (w3945:string)
            n2398 = Multiply(x=w3938, y=60000.0) -> (x*y=w3936:dbl)
            n2399 = VISA Write(VISA resource name=w3956, write buffer=w3945) -> (VISA resource name out=w3944:refnum<visa-resource-name>)  [unwired: 1 in, 2 out]
            n2400 = Concatenate Strings("cvolume" ("string"), "\r") -> (w3943:string)
            n2401 = VISA Write(VISA resource name=w3944, write buffer=w3943) -> (VISA resource name out=w3954:refnum<visa-resource-name>)  [unwired: 1 in, 2 out]
            n2402 = Concatenate Strings("irun" ("string"), "\r") -> (w3952:string)
            n2403 = VISA Write(VISA resource name=w3954, write buffer=w3952) -> (VISA resource name out=w3942:refnum<visa-resource-name>)  [unwired: 1 in, 2 out]
          }
          frame #1 {
            # "Have to wait until\nflow is done to reset\nrate"
            n2404 = Add(x=w3965, y=100.0) -> (x+y=w3964:dbl)
            n2405 = Wait (ms)(milliseconds to wait=w3964) -> ()  [unwired: 1 out]
          }
          frame #2 {
            # "reset flow rate to usual flow rate"
            n2406 = local read "Flow rate (uL/h)"() -> (w3977:dbl)
            n2407 = Number To Decimal String(number=w3977) -> (decimal integer string=w3975:string)  [unwired: 1 in]
            n2408 = Concatenate Strings("irate  " ("string"), w3975, " u/h" ("string"), "\r") -> (w3973:string)
            n2409 = VISA Write(VISA resource name=w3971, write buffer=w3973) -> (VISA resource name out=w3967:refnum<visa-resource-name>)  [unwired: 1 in, 2 out]
            n2410 = Concatenate Strings("cvolume" ("string"), "\r") -> (w3968:string)
            n2411 = VISA Write(VISA resource name=w3967, write buffer=w3968) -> ()  [unwired: 1 in, 3 out]
          }
        }
      }
      event "Flush Pump 3": Value Change {
        n2412 = event-data() -> ()  [unwired: 7 out]
        n2413 = flat-sequence {
          tunnel: w3978 -> [w3981]
          frame #0 {
            # "set paramaters (rate, volume) for flush, clear volume"
            n2414 = Number To Decimal String(number="Flush rate (uL/m) P3") -> (decimal integer string=w4003:string)  [unwired: 1 in]
            n2415 = local write "Inject Pump 3"(TRUE ("Inject Pump 3")) -> ()
            n2416 = Concatenate Strings("irate  " ("string"), w4003, " u/m" ("string"), "\r") -> (w4005:string)
            n2417 = VISA Write(VISA resource name=w3981, write buffer=w4005) -> (VISA resource name out=w4001:refnum<visa-resource-name>)  [unwired: 1 in, 2 out]
            n2418 = Reciprocal(x="Flush rate (uL/m) P3") -> (1/x=w3985:dbl)
            n2419 = Number To Decimal String(number="Volume (uL) P3") -> (decimal integer string=w3992:string)  [unwired: 1 in]
            n2420 = Multiply(x="Volume (uL) P3", y=w3985) -> (x*y=w3984:dbl)
            n2421 = Concatenate Strings("tvolume  " ("string"), w3992, " u" ("string"), "\r") -> (w3990:string)
            n2422 = Multiply(x=w3984, y=60.0) -> (x*y=→"HP3 Flush Time (s)":dbl)
            n2423 = VISA Write(VISA resource name=w4001, write buffer=w3990) -> (VISA resource name out=w3989:refnum<visa-resource-name>)  [unwired: 1 in, 2 out]
            n2424 = Concatenate Strings("cvolume" ("string"), "\r") -> (w3988:string)
            n2425 = VISA Write(VISA resource name=w3989, write buffer=w3988) -> (VISA resource name out=w3999:refnum<visa-resource-name>)  [unwired: 1 in, 2 out]
            n2426 = Concatenate Strings("irun" ("string"), "\r") -> (w3997:string)
            n2427 = VISA Write(VISA resource name=w3999, write buffer=w3997) -> ()  [unwired: 1 in, 3 out]
          }
          frame #1 {
            "Flushing P3" <- TRUE ("Flushing P3")
          }
        }
      }
      event "Flush Pump 1": Value Change {
        n2428 = event-data() -> ()  [unwired: 7 out]
        n2429 = flat-sequence {
          tunnel: [w4019] -> w4009
          tunnel: w4008 -> [w4012]
          tunnel: w4009 -> [_]
          frame #0 {
            # "set paramaters (rate, volume) for flush, clear volume"
            n2430 = local write "Inject Pump 1"(TRUE ("Inject Pump 1")) -> ()
            n2431 = Number To Decimal String(number="Flush rate (uL/m) P1") -> (decimal integer string=w4035:string)  [unwired: 1 in]
            n2432 = Concatenate Strings("irate  " ("string"), w4035, " u/m" ("string"), "\r") -> (w4037:string)
            n2433 = VISA Write(VISA resource name=w4012, write buffer=w4037) -> (VISA resource name out=w4033:refnum<visa-resource-name>)  [unwired: 1 in, 2 out]
            n2434 = Reciprocal(x="Flush rate (uL/m) P1") -> (1/x=w4016:dbl)
            n2435 = Number To Decimal String(number="Volume (uL) P1") -> (decimal integer string=w4024:string)  [unwired: 1 in]
            n2436 = Multiply(x="Volume (uL) P1", y=w4016) -> (x*y=w4015:dbl)
            n2437 = Concatenate Strings("tvolume  " ("string"), w4024, " u" ("string"), "\r") -> (w4022:string)
            n2438 = Multiply(x=w4015, y=60.0) -> (x*y=→"HP1 Flush Time (s)":dbl)
            n2439 = VISA Write(VISA resource name=w4033, write buffer=w4022) -> (VISA resource name out=w4021:refnum<visa-resource-name>)  [unwired: 1 in, 2 out]
            n2440 = Concatenate Strings("cvolume" ("string"), "\r") -> (w4020:string)
            n2441 = VISA Write(VISA resource name=w4021, write buffer=w4020) -> (VISA resource name out=w4031:refnum<visa-resource-name>)  [unwired: 1 in, 2 out]
            n2442 = Concatenate Strings("irun" ("string"), "\r") -> (w4029:string)
            n2443 = VISA Write(VISA resource name=w4031, write buffer=w4029) -> (VISA resource name out=w4019:refnum<visa-resource-name>)  [unwired: 1 in, 2 out]
          }
          frame #1 {
            "Flushing P1" <- TRUE ("Flushing P3")
          }
        }
      }
      event "Clear Volume": Value Change {
        n2444 = event-data() -> ()  [unwired: 7 out]
        n2445 = Concatenate Strings("cvolume" ("string"), "\r") -> (w4041:string)
        n2446 = VISA Write(VISA resource name=w4040, write buffer=w4041) -> ()  [unwired: 1 in, 3 out]
      }
      event "Clear Volume P3": Value Change {
        n2447 = event-data() -> ()  [unwired: 7 out]
        n2448 = Concatenate Strings("cvolume" ("string"), "\r") -> (w4047:string)
        n2449 = VISA Write(VISA resource name=w4046, write buffer=w4047) -> ()  [unwired: 1 in, 3 out]
        n2450 = local write "Clear Volume P3"(FALSE ("Clear Volume P3")) -> ()
      }
      event "Clear Volume P1": Value Change {
        n2451 = event-data() -> ()  [unwired: 7 out]
        n2452 = Concatenate Strings("cvolume" ("string"), "\r") -> (w4052:string)
        n2453 = local write "Clear Volume P1"(FALSE ("Clear Volume P1")) -> ()
        n2454 = VISA Write(VISA resource name=w4051, write buffer=w4052) -> ()  [unwired: 1 in, 3 out]
      }
      event "Display On P3": Value Change {
        n2455 = event-data() -> ()  [unwired: 7 out]
        n2456 = Select(t="dim 100", s="Display On P3", f="dim 0") -> (s? t:f=w4058:string)
        n2457 = Concatenate Strings(w4058, "\r") -> (w4060:string)
        n2458 = VISA Write(VISA resource name=w4055, write buffer=w4060) -> ()  [unwired: 1 in, 3 out]
      }
      event "Display On P1": Value Change {
        n2459 = event-data() -> ()  [unwired: 7 out]
        n2460 = Select(t="dim 100", s="Display On P1", f="dim 0") -> (s? t:f=w4065:string)
        n2461 = Concatenate Strings(w4065, "\r") -> (w4067:string)
        n2462 = VISA Write(VISA resource name=w4062, write buffer=w4067) -> ()  [unwired: 1 in, 3 out]
      }
      event "Retract Pump 3": Value Change {
        n2463 = event-data() -> ()  [unwired: 7 out]
        n2464 = local write "Retract Pump 3"(FALSE ("Retract Pump 3")) -> ()
        n2465 = case shown="True" "Retract Pump 3" {
          tunnel: w4069 -> [_ w4072]
          frame False {
          }
          frame True {
            n2466 = Number To Decimal String(number="Retract Rate (uL/m)") -> (decimal integer string=w4090:string)  [unwired: 1 in]
            n2467 = Concatenate Strings("wrate  " ("string"), w4090, " u/m" ("string"), "\r") -> (w4092:string)
            n2468 = VISA Write(VISA resource name=w4072, write buffer=w4092) -> (VISA resource name out=w4083:refnum<visa-resource-name>)  [unwired: 1 in, 2 out]
            n2469 = Number To Decimal String(number="Retract Vol 3 (uL)") -> (decimal integer string=w4085:string)  [unwired: 1 in]
            n2470 = Concatenate Strings("tvolume  " ("string"), w4085, " u" ("string"), "\r") -> (w4082:string)
            n2471 = VISA Write(VISA resource name=w4083, write buffer=w4082) -> (VISA resource name out=w4078:refnum<visa-resource-name>)  [unwired: 1 in, 2 out]
            n2472 = Concatenate Strings("cvolume" ("string"), "\r") -> (w4079:string)
            n2473 = VISA Write(VISA resource name=w4078, write buffer=w4079) -> (VISA resource name out=w4073:refnum<visa-resource-name>)  [unwired: 1 in, 2 out]
            n2474 = Concatenate Strings("wrun" ("string"), "\r") -> (w4074:string)
            n2475 = VISA Write(VISA resource name=w4073, write buffer=w4074) -> ()  [unwired: 1 in, 3 out]
          }
        }
      }
      event "Retract Pump 1": Value Change {
        n2476 = event-data() -> ()  [unwired: 7 out]
        n2477 = local write "Retract Pump 1"(FALSE ("Retract Pump 1")) -> ()
        n2478 = case shown="True" "Retract Pump 1" {
          tunnel: w4094 -> [_ w4099]
          frame False {
          }
          frame True {
            n2479 = local read "Retract Rate (uL/m)"() -> (w4097:dbl)
            n2480 = Number To Decimal String(number=w4097) -> (decimal integer string=w4115:string)  [unwired: 1 in]
            n2481 = Concatenate Strings("wrate  " ("string"), w4115, " u/m" ("string"), "\r") -> (w4117:string)
            n2482 = VISA Write(VISA resource name=w4099, write buffer=w4117) -> (VISA resource name out=w4109:refnum<visa-resource-name>)  [unwired: 1 in, 2 out]
            n2483 = Number To Decimal String(number="Retract Vol 1 (uL)") -> (decimal integer string=w4111:string)  [unwired: 1 in]
            n2484 = Concatenate Strings("tvolume  " ("string"), w4111, " u" ("string"), "\r") -> (w4108:string)
            n2485 = VISA Write(VISA resource name=w4109, write buffer=w4108) -> (VISA resource name out=w4105:refnum<visa-resource-name>)  [unwired: 1 in, 2 out]
            n2486 = Concatenate Strings("cvolume" ("string"), "\r") -> (w4106:string)
            n2487 = VISA Write(VISA resource name=w4105, write buffer=w4106) -> (VISA resource name out=w4100:refnum<visa-resource-name>)  [unwired: 1 in, 2 out]
            n2488 = Concatenate Strings("wrun" ("string"), "\r") -> (w4101:string)
            n2489 = VISA Write(VISA resource name=w4100, write buffer=w4101) -> ()  [unwired: 1 in, 3 out]
          }
        }
      }
      event "Flip Green Filter": Value Change {
        n2490 = event-data() -> ()  [unwired: 7 out]
        n2491 = Not(x="Flip Green Filter") -> (.not. x?=w4119:bool)
        n2492 = local write "Flip Green Filter"(w4119) -> ()
        n2493 = flat-sequence {
          tunnel: w4127 -> [w4132]
          tunnel: w4126 -> [w4131]
          tunnel: [w4129] -> w4124
          tunnel: [w4128] -> w4123
          tunnel: [w4134] -> w4122
          tunnel: w4124 -> [w4134]
          tunnel: [w4133] -> w4121
          tunnel: w4123 -> [w4133]
          tunnel: w4122 -> [w4138]
          tunnel: w4121 -> [w4137]
          tunnel: [w4136] -> w4125
          frame #0 {
            n2494 = xnode "Read/Write Control"("FPGA VI Reference In"=w4132, "error in"=w4131, "Green Filter Flipper"=TRUE) -> ("FPGA VI Reference Out"=w4129:T19, "error out"=w4128:errorcluster)
          }
          frame #1 {
            n2495 = Wait (ms)(milliseconds to wait=u32 100) -> ()  [unwired: 1 out]
          }
          frame #2 {
            n2496 = xnode "Read/Write Control"("FPGA VI Reference In"=w4138, "error in"=w4137, "Green Filter Flipper"=FALSE) -> ("error out"=w4136:errorcluster)  [unwired: 1 out]
          }
        }
      }
      event "Pump 1 contents", "Pump 3 contents": Value Change {
        n2497 = event-data() -> ()  [unwired: 7 out]
        n2498 = local read "Pump 1 contents"() -> (→"Pump 1 cont disp":string)
        n2499 = local read "Pump 3 contents"() -> (→"Pump 3 cont disp":string)
      }
